vi "Check Setting Visibility.vi"(11 "UI Data in":refnum<class "Settings UI.lvclass">) -> (0 "Channels Visible":bool, 1 "Advanced timing visible":bool, 2 "Conditional settings visible":bool, 3 "UI Data out":refnum<class "Settings UI.lvclass">)   [LabVIEW 2024, in "Output Sequencer.lvlib" / "Settings UI.lvclass"]
uses:
  Settings UI.lvclass
  Settings UI.lvclass/Settings UI.ctl
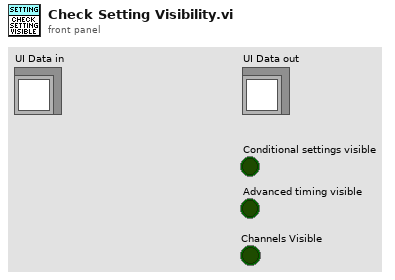
[diagram p1: front panel]
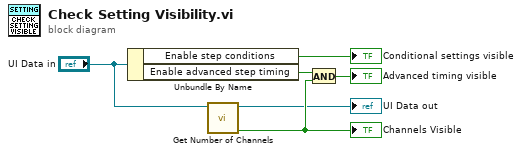
[diagram p0: block diagram]
diagram:
  n1 = Unbundle By Name("UI Data in") -> ("Enable step conditions"=→"Conditional settings visible":bool, "Enable advanced step timing"=w5:bool)
  n2 = call "Get Number of Channels.vi"("UI Data In"="UI Data in") -> ("Channels Defined"=w6:bool, "UI Data out"=→"UI Data out":refnum<class "Settings UI.lvclass">)  [unwired: 7 in, 2 out]
  "Channels Visible" <- w6
  n3 = And(x=w5, y=w6) -> (x .and. y?=→"Advanced timing visible":bool)
